vi "Advanced Calibrated True Rendering.vi"() -> ()   [LabVIEW 2020, in "examples.lvlib"]
doc: "Run an 3D Model based AR image pipeline which ensures that the 3D model is rendered as though it is a real object captured through a camera which introduces optical distortion."
uses:
  examples.lvlib
  ar/Chessboard Corner Info.ctl
  common/Object Point (Float).ctl
  common/Image Size (Integer).ctl
  common/Camera Parameters.ctl
  common/Camera Matrix.ctl
  common/Camera Distortion Coefficients.ctl
  ar/Image Distorter/Image Distorter.lvclass/Image Distorter.ctl
  ar/Point Correspondence Set.ctl
  common/Image Point (Float).ctl
  image/Image Read Size.ctl
  common/Termination Criteria/Termination Criteria.lvclass/Termination Criteria.ctl
  image/ARGB Colour.ctl
  image/New Image (Greyscale Preallocated).vi
  image/New Image (ARGB Preallocated).vi
  image/Read Image File (ARGB).vi
  ar/Find Chessboard Corners (Greyscale).vi
  ar/Solve PnP (IPPE).vi
  image/Copy Pixmap to Image (ARGB Flatten Mask).vi
  ar/Image Distorter/Distort Image (ARGB).vi
  image/In-Range (ARGB).vi
  image/Insert Image (ARGB with Greyscale Mask).vi
  image/Draw Image to Picture (Greyscale).vi
  image/Draw Image to Picture (ARGB).vi
  ar/Create Mesh form Verticies.vi
  ar/Apply Material Information.vi
  common/Break on NILRT-ARM32.vi
  image/New Image (Greyscale Preallocated).vi/6598b9e0-8a08-46f5-91fd-ca1b87217137.vi
  image/New Image (ARGB Preallocated).vi/3321fa97-f432-4e1e-8db9-a0df79aed21b.vi
  image/ARGB Colour to U32 Pixel Value.vi
  image/Read Image File (ARGB).vi/2358f293-6357-4b7a-bec3-c4e4d03be6e5.vi
  image/ARGBExtractChannel.vi
  ar/Find Chessboard Corners (Greyscale).vi/ca99938f-1423-42fb-b653-ffd1f73e2bb5.vi
  common/Termination Criteria/Get Values.vi
  ar/SolvePnPCore.vi
  ar/Rodrigues.vi
  ar/Rodrigues (RVec To RMat).vi
  ar/Transform Components to Transformation Matrix.vi
  <vilib>/Analysis/baseanly.llb/A x B.vi
  <vilib>/Analysis/baseanly.llb/Real A x B.vi
  image/Copy Pixmap to Image (ARGB Flatten Mask).vi/7d03ccf7-b889-4e8d-9f2a-57831e73dbde.vi
  ar/Image Distorter/Distort Image (ARGB).vi/ccc224f2-fea8-4097-85c8-c2b3fe04188f.vi
  image/In-Range (ARGB).vi/ffccc43a-a069-4092-9152-56f2c6e40fec.vi
  image/Invert In-Place (Greyscale Bitwise).vi/821d400d-177f-4d99-a785-a8086a4d8ddd.vi
  image/Insert Image (ARGB with Greyscale Mask).vi/5e3288c8-ee88-4cfe-89cf-31ceca475f5a.vi
  image/Draw Image to Picture (Greyscale).vi/9ae995ca-ccda-485c-89ac-02736fde3e8e.vi
  image/Draw Image to Picture (ARGB).vi/8cd07b1b-062e-4fe4-9e87-2eb3dc89fe0e.vi
  image/FixPixmap.vi
  image/Default8bitColourMap.vi
  <vilib>/Utility/error.llb/Error Cluster From Error Code.vi
  <vilib>/string/Create NI GUID.vi
  <vilib>/picture/3D Picture Control/Geometries/Create Mesh.vi
  <vilib>/picture/3D Picture Control/Object/Create Object (drawable).vi
  <vilib>/picture/3D Picture Control/Object/Set Material.vi
  <vilib>/Utility/libraryn.llb/Get File Extension.vi
  <vilib>/picture/jpeg.llb/Read JPEG File.vi
  <vilib>/picture/3D Picture Control/Helpers/Apply Texture.vi
  <vilib>/picture/3D Picture Control/Helpers/Apply Texture (no reference).vi
  <vilib>/picture/png.llb/Read PNG File.vi
  <vilib>/picture/bmp.llb/Read BMP File.vi
  <vilib>/picture/3D Picture Control/Object/Create Object (name).vi
  <vilib>/picture/3D Picture Control/Object/Add Object (no reference).vi
  <vilib>/picture/3D Picture Control/Object/Add Object (reference).vi
  <vilib>/Analysis/Matrix/Numeric/Conversions/Array To Matrix.vi
  <vilib>/Analysis/Matrix/Numeric/Conversions/Array To Matrix - RA2.vi
  ar/Image Distorter/Image Distorter.lvclass
  common/Termination Criteria/Termination Criteria.lvclass
  ar/ar.lvlib
  image/image.lvlib
  common/common.lvlib
  <vilib>/picture/3D Picture Control/NI_3D Picture Control.lvlib
  <vilib>/Utility/miscctls.llb/LVBoundsTypeDef.ctl
panel:
  out "Results":T1(array[cluster])
  out "3D Picture":refnum<vi>(3d-picture)
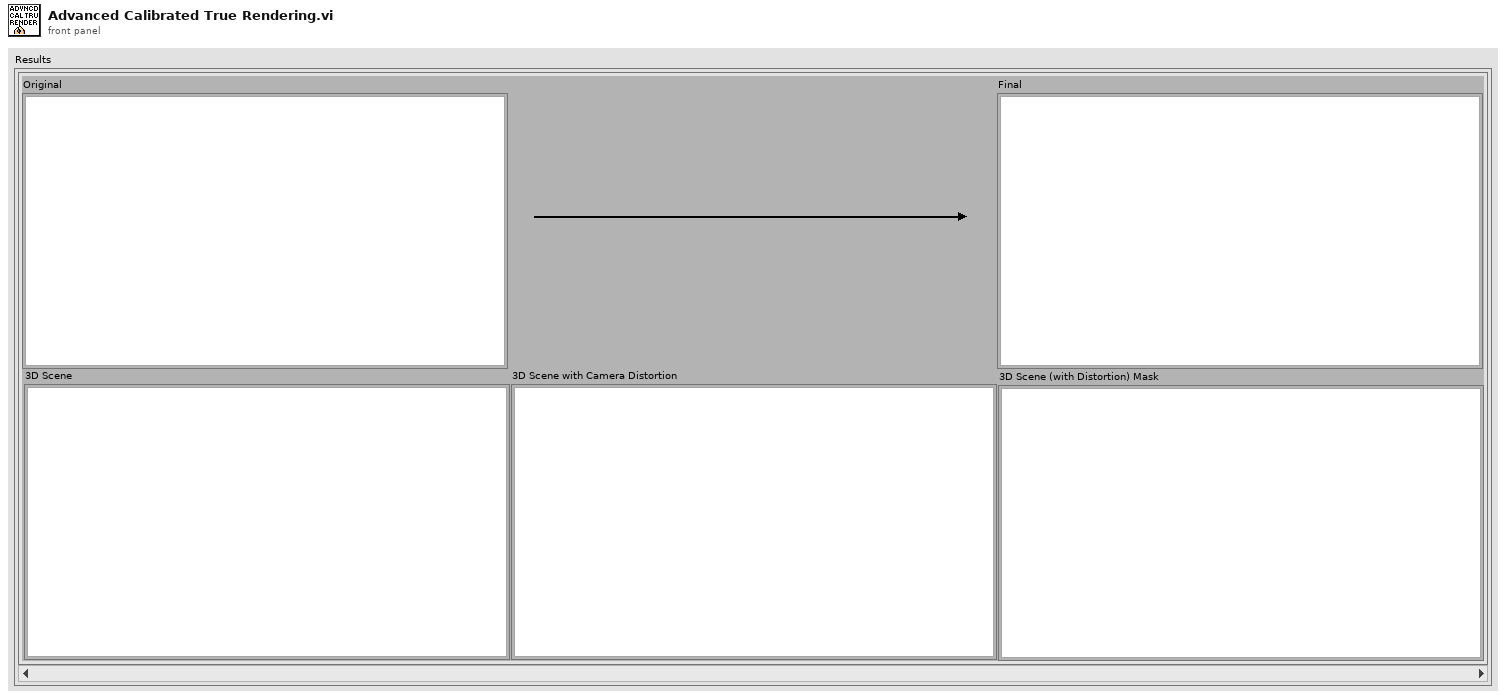
[diagram p1: front panel]
types:
  T1 = cluster{"Original":picture, "Final":picture, "3D Scene":picture, "3D Scene with Camera Distortion":picture, "3D Scene (with Distortion) Mask":picture}[]
  T2 = typedef "common.lvlib/Camera Parameters.ctl" = cluster{"Matrix":T3, "Distortion":T4}
  T3 = typedef "common.lvlib/Camera Matrix.ctl" = cluster{"m 0,0":dbl, "m 0,1":dbl, "m 0,2":dbl, "m 1,0":dbl, "m 1,1":dbl, "m 1,2":dbl, "m 2,0":dbl, "m 2,1":dbl, "m 2,2":dbl}
  T4 = typedef "common.lvlib/Camera Distortion Coefficients.ctl" = cluster{"k1":dbl, "k2":dbl, "p1":dbl, "p2":dbl, "k3":dbl, "k4":dbl, "k5":dbl, "k6":dbl, "s1":dbl, "s2":dbl, "s3":dbl, "s4":dbl, "tau x":dbl, "tau y":dbl}
  T5 = typedef "common.lvlib/Image Size (Integer).ctl" = cluster{"Width":u16, "Height":u16}
  T6 = typedef "LVBoundsTypeDef.ctl" = cluster{"Width":u32, "Height":u32}
  T7 = typedef "common.lvlib/Object Point (Float).ctl" = cluster{"x":dbl, "y":dbl, "z":dbl}
  T8 = typedef "ar.lvlib/Chessboard Corner Info.ctl" = cluster{"Points Per Row":u8, "Points Per Col":u8}
  T9 = cluster{"Points Per Row":i32, "Points Per Col":i32}
  T10 = typedef "image.lvlib/Image Read Size.ctl" = enum8{"FULL_SIZE", "REDUCED_2", "REDUCED_4", "REDUCED_8"}
  T11 = typedef "ar.lvlib/Point Correspondence Set.ctl" = cluster{"Object Points":T7[], "Image Points":T12[]}
  T12 = typedef "common.lvlib/Image Point (Float).ctl" = cluster{"x":dbl, "y":dbl}
  T13 = typedef "image.lvlib/Greyscale Image.ctl" = refnum<data-value>
  T14 = typedef "image.lvlib/ARGB Image.ctl" = refnum<data-value>
  T15 = typedef "ar.lvlib/Pose.ctl" = cluster{"rvec":T16, "tvec":T17}
  T16 = typedef "ar.lvlib/rvec.ctl" = cluster{"v0":dbl, "v1":dbl, "v2":dbl}
  T17 = typedef "ar.lvlib/tvec.ctl" = cluster{"x":dbl, "y":dbl, "z":dbl}
  T18 = typedef "image.lvlib/ARGB Colour.ctl" = cluster{"Alpha":u8, "RGB":u32}
  T19 = typedef "image.lvlib/In-Range Image Colour Range.ctl" = cluster{"Lower":u32, "Upper":u32}
  T20 = typedef "NI_Matrix.lvlib/RealMatrix.ctl" = dbl[][]
  T21 = typedef "imagedata.ctl" = cluster{"image type":i32, "image depth":i32, "image":u8[], "mask":u8[], "colors":u32[], "Rectangle":cluster{"left":i16, "top":i16, "right":i16, "bottom":i16}}
  T22 = cluster{"Picture":picture, "Picture":picture, "new picture":picture, "Picture":picture, "Picture":picture}
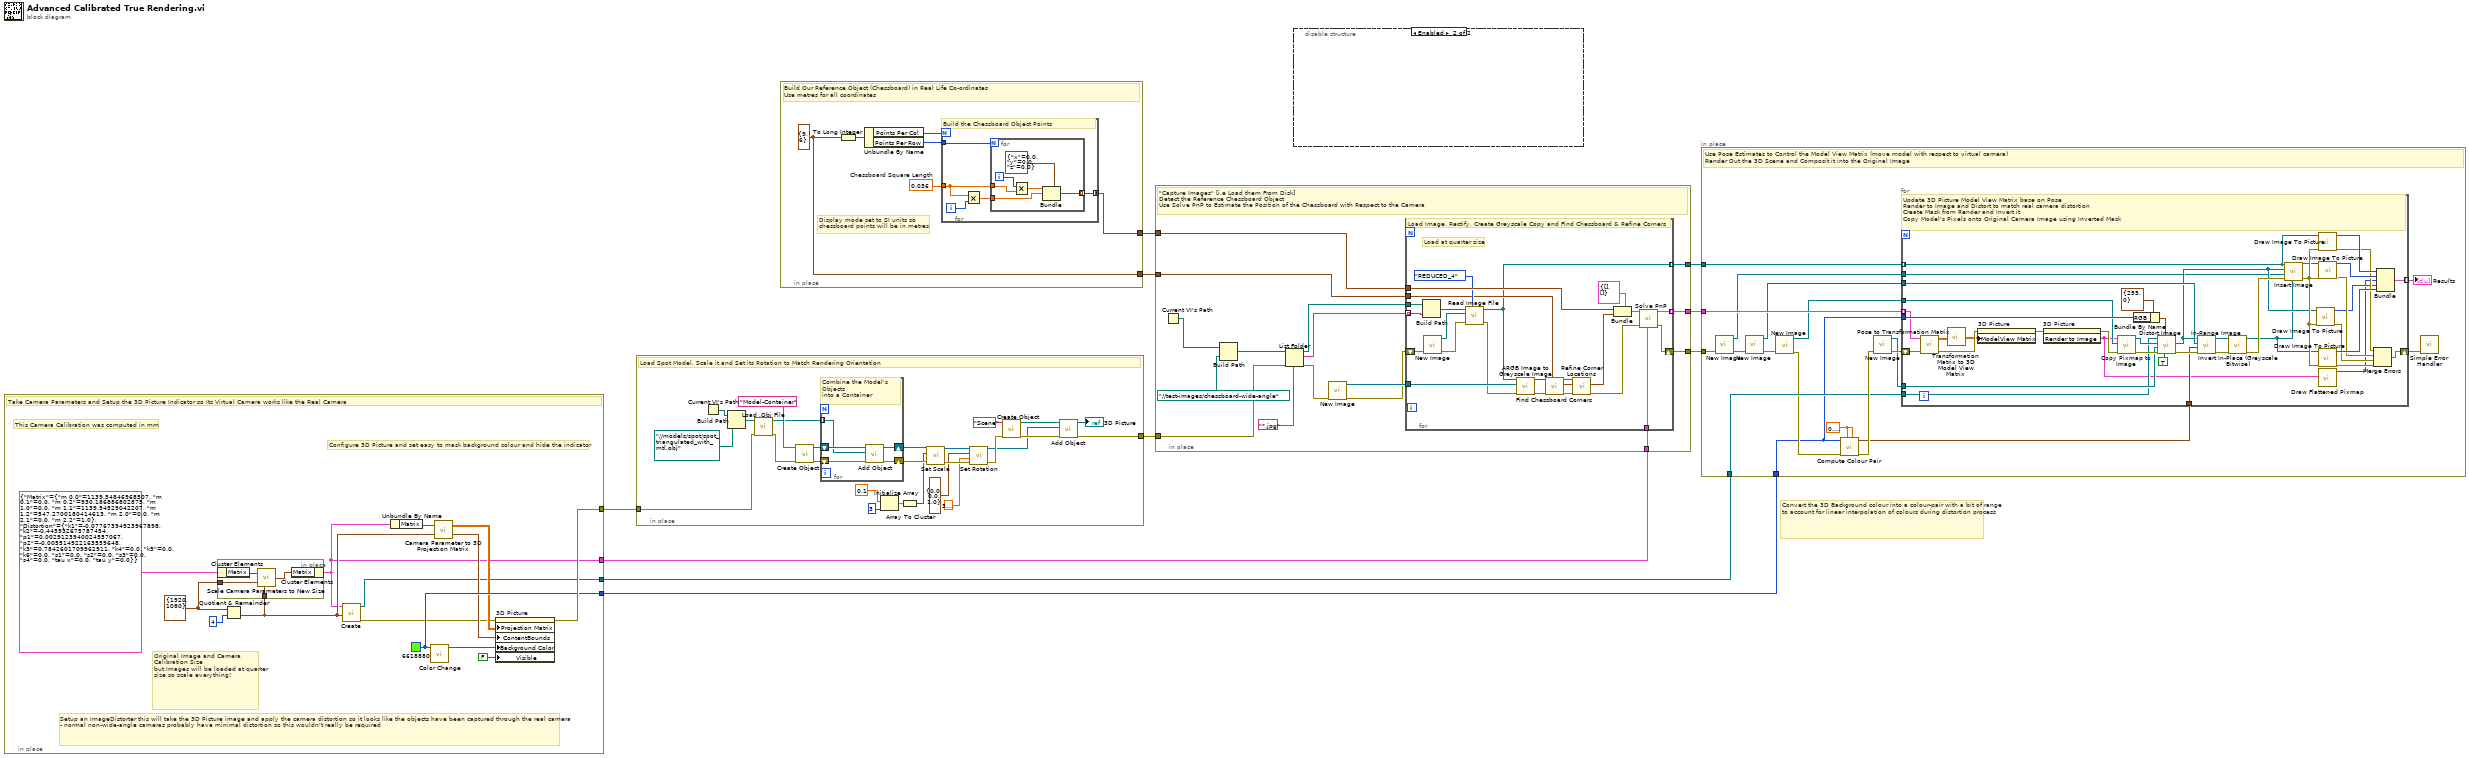
[diagram p0: block diagram]
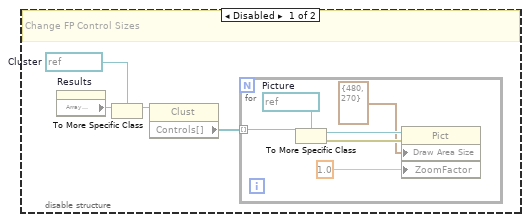
[diagram p2: hidden frame]
diagram:
  # "Convert the 3D Background colour into a colour-pair with a bit of range to account for linear interpolation of colours during distortion process"
  n1 = in-place {
    in-place-border: [w24] -> w9
    in-place-border: [w22] -> w6
    in-place-border: [w14] -> w2
    in-place-border: [w12] -> w1
    w17 = T5 {"Width"=1920, "Height"=1080} ("Size")
    w22 = u32 6618880 ("Color")
    # "Setup an ImageDistorter this will take the 3D Picture image and apply the camera distortion so it looks like the objects have been captured through the real camera\n- normal non-wide-angle cameras probably have minimal distortion so this wouldn't really be required"
    # "Original Image and Camera Calibration Size \nbut Images will be loaded at quarter size so scale everything!"
    # "Configure 3D Picture and set easy to mask background colour and hide the indicator"
    # "This Camera Calibration was computed in mm"
    # "Take Camera Parameters and Setup the 3D Picture Indicator so Its Virtual Camera works like the Real Camera"
    n2 = Quotient & Remainder(x=w17, y=u16 4) -> (floor(x/y)=w13:T5)  [unwired: 1 out]
    n3 = in-place {
      in-place-border: w13 -> [w28]
      in-place-border: w17 -> [w27]
      n4 = in-place-cluster #1(T2 {"Matrix"={"m 0,0"=1139.54846968507, "m 0,1"=0.0, "m 0,2"=930.186886802875, "m 1,0"=0.0, "m 1,1"=1139.94529042207, "m 1,2"=547.2700180414613, "m 2,0"=0.0, "m 2,1"=0.0, "m 2,2"=1.0}, "Distortion"={"k1"=-0.07767394923967898, "k2"=-0.445932675787454, "p1"=0.0029123940024557067, "p2"=-0.005514922163559648, "k3"=0.7842601709962911, "k4"=0.0, "k5"=0.0, "k6"=0.0, "s1"=0.0, "s2"=0.0, "s3"=0.0, "s4"=0.0, "tau x"=0.0, "tau y"=0.0}} ("Camera Parameters")) -> ("Matrix"=w26:T3)
      n5 = call "Scale Camera Parameters to New Size.vi"("New Size"=w28, "Current Size"=w27, "Camera Matrix"=w26) -> ("Scaled Camera Matrix"=w25:T3)
      n6 = in-place-cluster #1("Matrix"=w25) -> (w12:T2)
    }
    n7 = call "Create.vi"("Image Size"=w13, "Camera Parameters"=w12) -> ("error out"=w15:errorcluster, "Image Distorter"=w14:refnum<class "Image Distorter.lvclass">)  [unwired: 8 in]
    n8 = Unbundle By Name(w12) -> ("Matrix"=w16:T3)
    n9 = call <vilib>:"Color Change.vi"("Color"=w22) -> ("RGBA"=w23:cluster{"R":sgl, "G":sgl, "B":sgl, "A":sgl})  [unwired: 10 in]
    n10 = call "Camera Parameter to 3D Projection Matrix.vi"("Size"=w13, "Camera Matrix"=w16) -> ("Bounds"=w19:T6, "3D-Picture Projection Matrix"=w18:sgl[][])  [unwired: 2 in]
    n11 = property on="3D Picture" class="SceneGraphDisp (strict)"(error in=w15, "Projection Matrix"=w18, "ContentBounds"=w19, "Background Color"=w23, "Visible"=FALSE) -> (error out=w24:errorcluster)  [unwired: 1 in, 1 out]
  }
  n12 = in-place {
    in-place-border: [w49] -> w10
    in-place-border: w9 -> [w48]
    # "Load Spot Model, Scale it and Set its Rotation to Match Rendering Orientation"
    n13 = Current VI's Path() -> (path=w54:path)
    n14 = Build Path(base path=w54, name or relative path=path "../../models/spot/spot_triangulated_with_mtl.obj" ("Path")) -> (appended path=w53:path)
    n15 = call "Load .Obj File.vi"("error in (no error)"=w48, "Object Model Path"=w53) -> ("error out"=w46:errorcluster, "Objects"=w42:refnum<vi>[])  [unwired: 7 in, 1 out]
    n16 = call-poly <vilib>:"Create Object.vi"("error in (no error)"=w46, "Name"="Model-Container") -> ("error out"=w44:errorcluster, "Scene:New Object"=w43:refnum<vi>)  [unwired: 8 in]
    n17 = for {
      tunnel: w42 -> [w57] mode=indexing
      shift-right: [w56] -> w41
      shift-left: w43 -> [w58]
      shift-right: [w55] -> w40
      shift-left: w44 -> [w59]
      # "Combine the Model's Objects\ninto a Container"
      n18 = call-poly <vilib>:"Add Object.vi"("error in (no error)"=w59, "New Object In"=w57, "Scene Object In"=w58) -> ("error out"=w55:errorcluster, "Scene Object Out"=w56:refnum<vi>)  [unwired: 7 in]
    }
    n19 = Initialize Array(0.1, 3 ("dimension size")) -> (w36:dbl[])
    n20 = Array To Cluster(array=w36) -> (cluster=w35:cluster{"[0]":dbl, "[1]":dbl, "[2]":dbl})
    n21 = call <vilib>:"Set Scale.vi"("error in (no error)"=w40, "Scale"=w35, "Scene Object"=w41) -> ("error out"=w39:errorcluster, "Scaled Object"=w33:refnum<vi>)  [unwired: 7 in]
    n22 = call <vilib>:"Set Rotation.vi"("error in (no error)"=w39, "Angle"=3.141592653589793, "Axis"=cluster{"X":sgl, "Y":sgl, "Z":sgl} {"X"=0.0, "Y"=0.0, "Z"=1.0}, "Scene Object"=w33) -> ("error out"=w34:errorcluster, "Rotated Scene Object"=w32:refnum<vi>)  [unwired: 6 in]
    n23 = call-poly <vilib>:"Create Object.vi"("error in (no error)"=w34, "Name"="Scene") -> ("error out"=w50:errorcluster, "Scene:New Object"=w51:refnum<vi>)  [unwired: 8 in]
    n24 = call-poly <vilib>:"Add Object.vi"("error in (no error)"=w50, "New Object In"=w32, "Scene Object In"=w51) -> ("error out"=w49:errorcluster, "Scene Object Out"=→"3D Picture":refnum<vi>)  [unwired: 6 in, 1 out]
  }
  n25 = in-place {
    in-place-border: [w61] -> w5
    in-place-border: [w63] -> w4
    w60 = 0.036  # Chessboard Square Length
    w61 = T8 {"Points Per Row"=9, "Points Per Col"=6} ("Chessboard Corners Info")
    # "Display mode set to SI units so \nchessboard points will be in metres"
    # "Build Our Reference Object (Chessboard) in Real Life Co-ordinates\nUse metres for all coordinates"
    n26 = To Long Integer(number=w61) -> (32bit integer=w62:T9)
    n27 = Unbundle By Name(w62) -> ("Points Per Col"=w65:i32, "Points Per Row"=w64:i32)
    n28 = for {
      N: w65 -> [_]
      tunnel: w64 -> [w70]
      tunnel: w60 -> [w68]
      tunnel: [w66] -> w63 mode=concatenating
      i -> [w69]
      # "Build the Chessboard Object Points"
      n29 = Multiply(x=w68, y=w69) -> (x*y=w67:dbl)
      n30 = for {
        N: w70 -> [_]
        tunnel: w68 -> [w76]
        tunnel: w67 -> [w72]
        tunnel: [w71] -> w66 mode=indexing
        i -> [w75]
        n31 = Multiply(x=w75, y=w76) -> (x*y=w73:dbl)
        n32 = Bundle(cluster=T7 {"x"=0.0, "y"=0.0, "z"=0.0} ("Object Point"), "x"=w73, "y"=w72) -> (w71:T7)  [unwired: 1 in]
      }
    }
  }
  n33 = in-place {
    in-place-border: w10 -> [w86]
    in-place-border: [w85] -> w8
    in-place-border: [w84] -> w7
    in-place-border: w5 -> [w83]
    in-place-border: w4 -> [w82]
    in-place-border: [w81] -> w3
    in-place-border: w1 -> [w77]
    # "\"Capture Images\" [i.e Load them From Disk]\nDetect the Reference Chessboard Object\nUse Solve PnP to Estimate the Position of the Chessboard with Respect to the Camera"
    n34 = Current VI's Path() -> (path=w79:path)
    n35 = Build Path(base path=w79, name or relative path=path "../../test-images/chessboard-wide-angle") -> (appended path=w90:path)
    n36 = List Folder(path=w90, pattern="*.jpg", error in=w86) -> (path out=w89:path, filenames=w87:string[], error out=w88:errorcluster)  [unwired: 1 in, 1 out]
    n37 = call-poly "New Image.vi"("error in (no error)"=w88) -> ("error out"=w80:errorcluster, "Greyscale Image"=w92:T13)  [unwired: 9 in]
    n38 = for {
      tunnel: w89 -> [w115]
      tunnel: w87 -> [w114] mode=indexing
      shift-right: [w103] -> w84
      shift-left: w80 -> [w97]
      tunnel: w83 -> [w98]
      tunnel: w82 -> [w112]
      tunnel: [w100] -> w85 mode=indexing
      tunnel: w92 -> [w108]
      tunnel: [w95] -> w81 mode=indexing
      tunnel: w77 -> [w93]
      # "Load at quarter size"
      # "Load Image, Rectify, Create Greyscale Copy and Find Chessboard & Refine Corners"
      n39 = Build Path(base path=w115, name or relative path=w114) -> (appended path=w113:path)
      n40 = call-poly "New Image.vi"() -> ("ARGB Image"=w94:T14)  [unwired: 10 in, 1 out]
      n41 = call-poly "Read Image File.vi"("Image Read Size (Default: FULL_SIZE)"=Image_Read_Size."REDUCED_4", "error in (no error)"=w97, "ARGB Image Destination in"=w94, "Filepath"=w113) -> ("error out"=w96:errorcluster, "ARGB Image Destination"=w95:T14)  [unwired: 6 in]
      n42 = call "ARGB Image to Greyscale Image.vi"("error in (no error)"=w96, "Greyscale Image Destination in"=w108, "ARGB Image Source in"=w95) -> ("error out"=w105:errorcluster, "Greyscale Image Destination"=w107:T13)  [unwired: 7 in]
      n43 = call-poly "Find Chessboard Corners.vi"("Chessboard Corners Info"=w98, "error in (no error)"=w105, "Greyscale Image in"=w107) -> ("error out"=w111:errorcluster, "Points"=w110:T12[], "Greyscale Image"=w106:T13)  [unwired: 6 in]
      n44 = call "Refine Corner Locations.vi"("error in (no error)"=w111, "Points in"=w110, "Greyscale Image in"=w106) -> ("error out"=w104:errorcluster, "Points out"=w109:T12[])  [unwired: 6 in, 1 out]
      n45 = Bundle(cluster=T11 {"Object Points"=[], "Image Points"=[]} ("Point Correspondence Set"), "Object Points"=w112, "Image Points"=w109) -> (w101:T11)
      n46 = call-poly "Solve PnP.vi"("Camera Parameters"=w93, "error in (no error)"=w104, "Point Correspondence Set"=w101) -> ("error out"=w103:errorcluster, "Pose"=w100:T15)  [unwired: 7 in]
    }
  }
  n47 = disable-structure shown="Enabled" {
    frame Disabled {
      w117 = refnum<vi> refnum  # Cluster
      # "Change FP Control Sizes"
      n48 = property on="Results" class="Arr (strict)"() -> ("Array Element"=w119:refnum<vi>)  [unwired: 2 in, 2 out]
      n49 = To More Specific Class(target class=w117, reference=w119) -> (specific class reference=w118:refnum<vi>)  [unwired: 1 in, 1 out]
      n50 = property class="Clust"(reference=w118) -> ("Controls[]"=w116:refnum<vi>[])  [unwired: 1 in, 2 out]
      n51 = for {
        tunnel: w116 -> [w125] mode=indexing
        w124 = refnum<vi> refnum  # Picture
        n52 = To More Specific Class(target class=w124, reference=w125) -> (specific class reference=w123:refnum<vi>, error out=w122:errorcluster)  [unwired: 1 in]
        n53 = property class="Pict"(reference=w123, error in=w122, "Draw Area Size"=T6 {"Width"=480, "Height"=270}, "ZoomFactor"=sgl 1.0 ("Zoom Factor")) -> ()  [unwired: 2 out]
      }
    }
    frame Enabled {
    }
  }
  n54 = in-place {
    in-place-border: w8 -> [w143]
    in-place-border: w7 -> [w142]
    in-place-border: w6 -> [w127]
    in-place-border: w3 -> [w134]
    in-place-border: w2 -> [w129]
    w130 = sgl 0.7 ("Fractional_Scale")
    # "Use Pose Estimates to Control the Model View Matrix (move model with respect to virtual camera)\nRender Out the 3D Scene and Composit it into the Original Image"
    n55 = call-poly "New Image.vi"("error in (no error)"=w142) -> ("error out"=w139:errorcluster, "ARGB Image"=w138:T14)  [unwired: 9 in]
    n56 = call-poly "New Image.vi"("error in (no error)"=w139) -> ("error out"=w136:errorcluster, "Greyscale Image"=w141:T13)  [unwired: 9 in]
    n57 = call-poly "New Image.vi"("error in (no error)"=w136) -> ("error out"=w128:errorcluster, "ARGB Image"=w140:T14)  [unwired: 9 in]
    n58 = call "Compute Colour Pair.vi"("Fractional Scale Upper"=w130, "Fractional Scale Lower"=w130, "error in (no error)"=w128, "Starting Colour"=w127) -> ("error out"=w132:errorcluster, "Colour Pair"=w131:T19)  [unwired: 6 in]
    n59 = call-poly "New Image.vi"("error in (no error)"=w132) -> ("error out"=w135:errorcluster, "ARGB Image"=w133:T14)  [unwired: 9 in]
    n60 = for {
      tunnel: w143 -> [w145] mode=indexing
      tunnel: w141 -> [w175]
      tunnel: w140 -> [w151]
      tunnel: w138 -> [w146]
      shift-right: [w163] -> w137
      shift-left: w135 -> [w179]
      tunnel: w131 -> [w156]
      tunnel: [w162] -> w126 mode=indexing
      tunnel: w134 -> [w144] mode=indexing
      tunnel: w133 -> [w158]
      tunnel: w129 -> [w157]
      tunnel: w127 -> [w152]
      # "Update 3D Picture Model View Matrix base on Pose\nRender to Image and Distort to match real camera distortion\nCreate Mask from Render and Invert it\nCopy Model's Pixels onto Original Camera Image using Inverted Mask"
      n61 = call "Pose to Transformation Matrix.vi"("error in (no error)"=w179, "Pose"=w145) -> ("error out"=w180:errorcluster, "4x4 Transformation Matrix"=w173:T20)  [unwired: 8 in]
      n62 = call "Transformation Matrix to 3D Model View Matrix.vi"("4x4 Transformation Matrix"=w173) -> ("3D-Control Model Matrix"=w178:T20)
      n63 = property on="3D Picture" class="SceneGraphDisp (strict)"(error in=w180, "ModelView Matrix"=w178) -> (error out=w177:errorcluster)  [unwired: 1 in, 1 out]
      n64 = invoke on="3D Picture" class="SceneGraphDisp (strict)" method="Render to Image"(error in=w177) -> (error out=w181:errorcluster, "Get Image"=w147:T21)  [unwired: 2 in, 1 out]
      n65 = call-poly "Copy Pixmap to Image.vi"("error in (no error)"=w181, "ARGB Image Destination in"=w151, "Pixmap Image Data"=w147) -> ("error out"=w176:errorcluster, "ARGB Image Destination"=w160:T14)  [unwired: 7 in]
      n66 = Bundle By Name(cluster=T18 {"Alpha"=255, "RGB"=0} ("ARGB Colour (Default: Black)"), "RGB"=w152) -> (w153:T18)
      n67 = call-poly "Distort Image.vi"("Use Fixed Point Remapping (Default: False)"=TRUE, "ARGB Colour (Default: Black)"=w153, "error in (no error)"=w176, "ARGB Image Destination in"=w158, "ARGB Image Source in"=w160, "Image Distorter in"=w157) -> ("error out"=w161:errorcluster, "ARGB Image Destination"=w159:T14)  [unwired: 3 in, 1 out]
      n68 = call-poly "In-Range Image.vi"("error in (no error)"=w161, "In-Range Image Colour Range"=w156, "In-Range-Result in"=w175, "ARGB Image Source in"=w159) -> ("error out"=w171:errorcluster, "In-Range-Result"=w172:T13)  [unwired: 6 in]
      n69 = call "Invert In-Place (Greyscale Bitwise).vi"("error in (no error)"=w171, "Greyscale Image to Invert in Place in"=w172) -> ("error out"=w182:errorcluster, "Greyscale Image"=w155:T13)  [unwired: 8 in]
      n70 = call-poly "Insert Image.vi"("Greyscale Image Mask in"=w155, "error in (no error)"=w182, "ARGB Image Destination in"=w146, "ARGB Image Child in"=w159, "ARGB Image Parent in"=w144) -> ("error out"=w183:errorcluster, "ARGB Image Destination"=w174:T14)  [unwired: 5 in]
      n71 = call-poly "Draw Image To Picture.vi"("error in (no error)"=w183, "ARGB Image Source in"=w159) -> ("error out"=w166:errorcluster, "Picture"=w150:picture)  [unwired: 8 in]
      n72 = call-poly "Draw Image To Picture.vi"("error in (no error)"=w183, "ARGB Image Source in"=w144) -> ("error out"=w165:errorcluster, "Picture"=w170:picture)  [unwired: 8 in]
      n73 = call-poly "Draw Image To Picture.vi"("error in (no error)"=w183, "Greyscale Image Source in"=w155) -> ("error out"=w167:errorcluster, "Picture"=w168:picture)  [unwired: 8 in]
      n74 = call <vilib>:"Draw Flattened Pixmap.vi"("image data"=w147) -> ("new picture"=w149:picture)  [unwired: 8 in]
      n75 = call-poly "Draw Image To Picture.vi"("error in (no error)"=w183, "ARGB Image Source in"=w174) -> ("error out"=w164:errorcluster, "Picture"=w169:picture)  [unwired: 8 in]
      n76 = Merge Errors(w165, w164, w166, w167) -> (w163:errorcluster)
      n77 = Bundle("Picture"=w170, "Picture"=w169, "new picture"=w149, "Picture"=w150, "Picture"=w168) -> (w162:T22)  [unwired: 1 in]
    }
    "Results" <- w126
    n78 = call <vilib>:"Simple Error Handler.vi"("error in (no error)"=w137) -> ()  [unwired: 4 in, 5 out]
  }
